vi "p00 Simple Math.vi"() -> ()   [LabVIEW 2025]
panel:
  out "x*y":i16
  out "x-y":i16
  out "x+y":i16
  in  "y":i16
  in  "x":i16
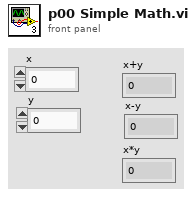
[diagram p1: front panel]
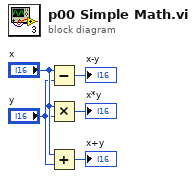
[diagram p0: block diagram]
diagram:
  n1 = Subtract(x="x", y="y") -> (x-y=→"x-y":i16)
  n2 = Multiply(x="x", y="y") -> (x*y=→"x*y":i16)
  n3 = Add(x="x", y="y") -> (x+y=→"x+y":i16)
